vi "Actor Core.vi"(8 "error in":errorcluster caption="错误输入", 11 "TPP demo V2 in":refnum<class "TPP demo V2.lvclass"> caption="操作者输入") -> (0 "error out":errorcluster caption="错误输出", 3 "Actor out":refnum<class "Actor.lvclass"> caption="操作者输出")   [LabVIEW 2017, in "TPP demo V2.lvlib" / "TPP demo V2.lvclass"]
doc: "(<B>Filename</B>: Actor Framework.lvlib:Actor.lvclass:Actor Core.vi)\n\nReceives messages to the actor, reacts to them, and initiates any error handling that may shut the actor down.\n\nDescendant classes may override this VI to append parallel tasks for the actor to complete while it handles messages.使用调用父方法节点实现重写。"
uses:
  TPP demo V2.lvclass
  E:/Program Files (x86)/National Instruments/LabVIEW 2017/vi.lib/ActorFramework/Actor/Actor.lvclass
  <vilib>/ActorFramework/Actor/Actor.lvclass
  Programmatic Controller/Programmatic Controller.lvclass
  <vilib>/ActorFramework/Actor/Actor.lvclass/Actor.ctl
  <vilib>/ActorFramework/Message Enqueuer/Message Enqueuer.lvclass/Message Enqueuer.ctl
  TPP demo V2.lvclass/TPP demo V2.ctl
  <vilib>/ActorFramework/Message Enqueuer/Init from Existing Queue.vi
  <vilib>/ActorFramework/Message Enqueuer/Enqueue.vi
  <vilib>/ActorFramework/Stop Msg/Stop Msg.lvclass
  E:/Program Files (x86)/National Instruments/LabVIEW 2017/vi.lib/ActorFramework/Message/Message.lvclass
  <vilib>/ActorFramework/Message Priority Queue/Priority Enqueue.vi
  <vilib>/ActorFramework/Message Enqueuer/Message Enqueuer.lvclass
panel:
  out "事件记录":string
  in  "停止":bool
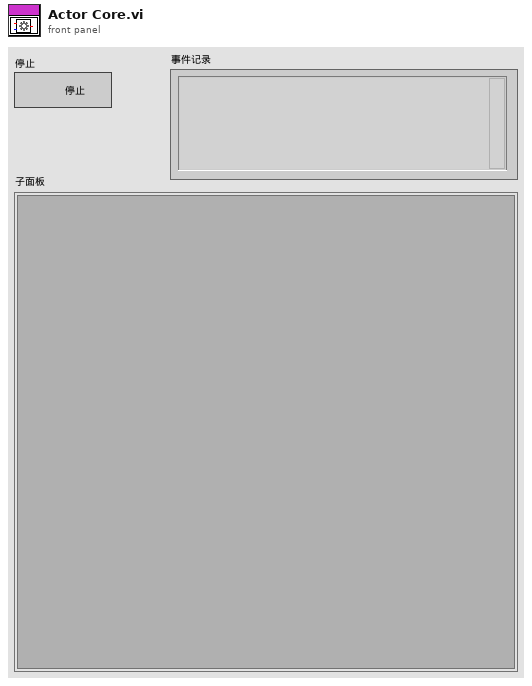
[diagram p1: front panel]
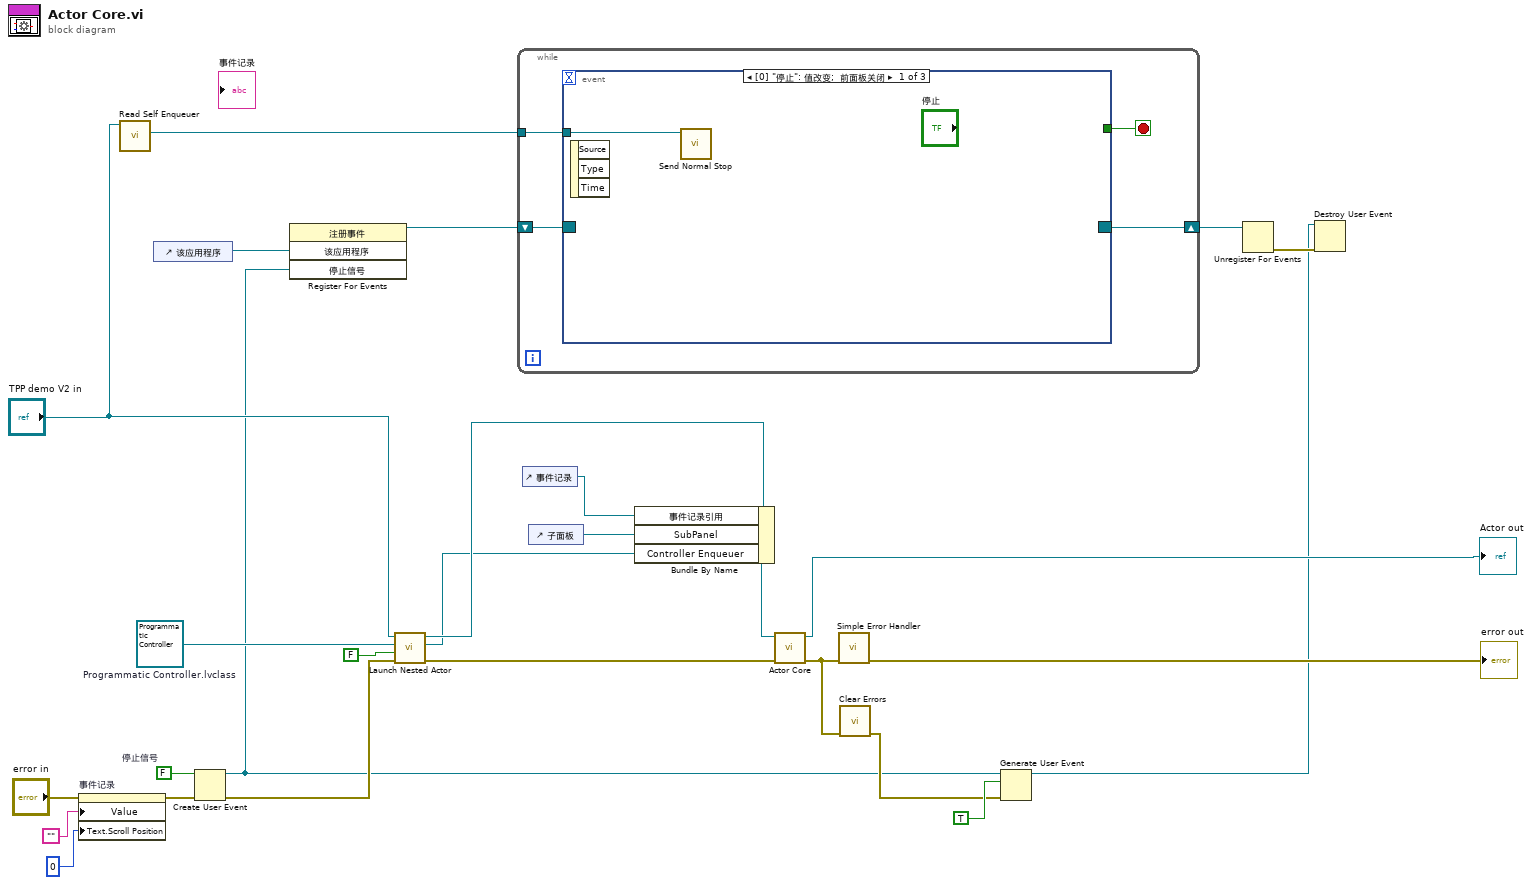
[diagram p0: block diagram]
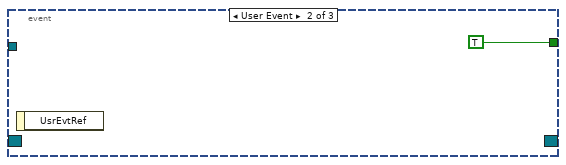
[diagram p2: hidden frame]
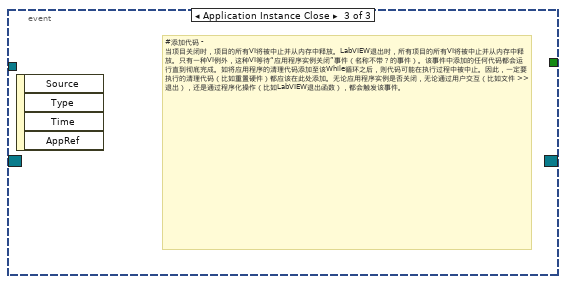
[diagram p3: hidden frame]
diagram:
  w8 = refnum<class "Programmatic Controller.lvclass"> refnum  # Programmatic Controller.lvclass
  w16 = FALSE  # 停止信号
  n1 = property on="事件记录" class="Str"(error in="error in", "Value"="", "Text.Scroll Position"=u32 0 ("文本.滚动条位置")) -> (error out=w15:errorcluster)  [unwired: 1 in, 1 out]
  n2 = call <vilib>:"Read Self Enqueuer.vi"("Actor"="TPP demo V2 in") -> ("Self Enqueuer"=w26:refnum<class "Message Enqueuer.lvclass">)  [unwired: 10 in]
  n3 = control-ref of="该应用程序"() -> (w6:refnum<vi>)
  n4 = Create User Event(user event datatype=w16, error in=w15) -> (user event=w7:refnum<user-event>, error out=w14:errorcluster)
  n5 = register-events(w6, w7) -> (reference out=w5:refnum<event-registration>)  [unwired: 2 in, 1 out]
  n6 = call <vilib>:"Launch Nested Actor.vi"("error in (no error)"=w14, "Auto-stop? (T)"=FALSE, "Nested Actor"=w8, "Caller Actor in"="TPP demo V2 in") -> ("error out"=w25:errorcluster, "Nested Actor's Enqueuer"=w9:refnum<class "Message Enqueuer.lvclass">, "Caller Actor out"=w24:refnum<class "TPP demo V2.lvclass">)  [unwired: 5 in]
  n7 = while {
    tunnel: w26 -> [w31]
    shift-right: [w28] -> w4
    shift-left: w5 -> [w29]
    stop <- w30 stop-if-true
    n8 = event shown="[0] \"停止\": 值改变;  前面板关闭" {
      selector: w29 -> [_ _ _]
      dyn-events: [_ _ _] -> w28
      timeout: _ -> [_ _ _]
      tunnel: w31 -> [w32 _ _]
      tunnel: [_ TRUE _] -> w30
      event "停止": Value Change; Panel Close {
        n9 = event-data() -> ()  [unwired: 1 in, 3 out]
        n10 = call <vilib>:"Send Normal Stop.vi"("Message Enqueuer"=w32) -> ()  [unwired: 10 in, 1 out]
      }
      event User Event {
        n11 = event-data() -> ()  [unwired: 1 in, 1 out]
      }
      event Application Instance Close {
        # "#添加代码 - 当项目关闭时，项目的所有VI将被中止并从内存中释放。LabVIEW退出时，所有项目的所有VI将被中止并从内存中释放。只有一种VI例外，这种VI等待“应用程序实例关闭”事件（名称不带？的事件）。该事件中添加的任何代码都会运行直到彻底完成。如将应用程序的清理代码添加至该While循环之后，则代码可能在执行过程中被中止。因此，一定要执行的清理代码（比如重置硬件）都应该在此处添加。无论应用程序实例是否关闭，无论通过用户交互（比如文件 >> 退出），还是通过程序化操作（比如LabVIEW退出函数），都会触发该事件。"
        n12 = event-data() -> ()  [unwired: 1 in, 4 out]
      }
    }
  }
  n13 = control-ref of="事件记录"() -> (w23:refnum<vi>)
  n14 = control-ref of="子面板"() -> (w17:refnum<vi>)
  n15 = Bundle By Name(cluster=w24, "事件记录引用"=w23, "SubPanel"=w17, "Controller Enqueuer"=w9) -> (w22:refnum<class "TPP demo V2.lvclass">)
  n16 = call-parent "Actor Core.vi"("error in"=w25, "Actor in"=w22) -> ("error out"=w11:errorcluster, "Actor out"=→"Actor out":refnum<class "Actor.lvclass">)  [unwired: 8 in]
  n17 = call <vilib>:"Simple Error Handler.vi"("error in (no error)"=w11) -> ("error out"=→"error out":errorcluster)  [unwired: 4 in, 4 out]
  n18 = call <vilib>:"Clear Errors.vi"("error in (no error)"=w11) -> ("error out"=w10:errorcluster)  [unwired: 5 in, 1 out]
  n19 = Generate User Event(user event=w7, event data cluster=TRUE ("值(信号)"), error in=w10) -> (user event out=w2:refnum<user-event>)  [unwired: 1 in, 1 out]
  n20 = Unregister For Events(event registration refnum=w4) -> (error out=w3:errorcluster)  [unwired: 1 in]
  n21 = Destroy User Event(user event=w2, error in=w3) -> ()  [unwired: 1 out]
